vi "Noise-Create.vi"(4 "Rep Num":i32, 6 "Name":string, 8 "error in (no error)":errorcluster, 9 "Npts":i32, 10 "Sampling Rate (Hz)":dbl, 11 "Noise Params":T1) -> (0 "error out":errorcluster, 2 "Waveform":dbl[](array[numeric]), 3 "Noise Params (out)":T1)   [LabVIEW 2020]
uses:
  Noise Params.ctl
  Noise-Globals.vi
  <vilib>/Analysis/NI_AALBase.lvlib
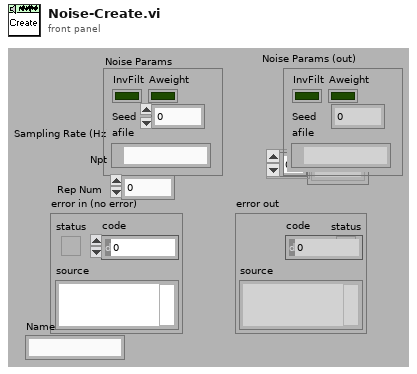
[diagram p1: front panel]
types:
  T1 = typedef "Noise Params.ctl" = cluster{"InvFilt":bool, "Noise":dbl[], "CurPt":i32, "Aweight":bool, "Seed":i32, "afile":path}
  T2 = enum16{"Clear", "Set data", "Reset index", "Get data"}
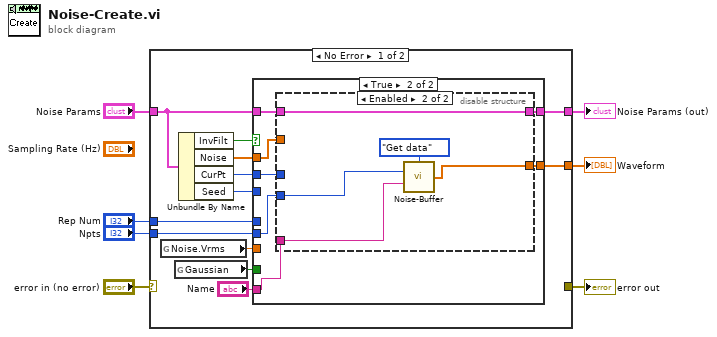
[diagram p0: block diagram]
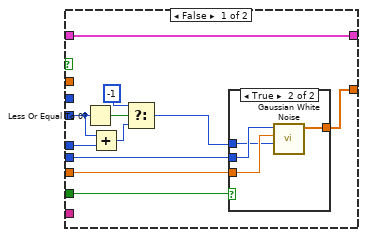
[diagram p2: hidden frame]
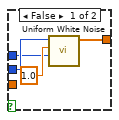
[diagram p3: hidden frame]
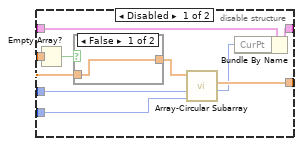
[diagram p4: hidden frame]
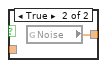
[diagram p5: hidden frame]
diagram:
  n1 = case shown="No Error" "error in (no error)" {
    selector: "error in (no error)" -> [_ w63]
    tunnel: "Npts" -> [w19 _]
    tunnel: [w18 _] -> w6
    tunnel: [_ w63] -> w4
    tunnel: [w15 w62] -> w2
    tunnel: "Noise Params" -> [w16 w62]
    tunnel: "Rep Num" -> [w9 _]
    frame No Error {
      n2 = global read "Noise-Globals.vi" "Noise.Vrms"() -> (w13:dbl)
      n3 = global read "Noise-Globals.vi" "Gaussian"() -> (w14:bool)
      n4 = Unbundle By Name(w16) -> ("InvFilt"=w8:bool, "Noise"=w12:dbl[], "CurPt"=w17:i32, "Seed"=w10:i32)
      n5 = case shown="True" w8 {
        tunnel: w19 -> [w22 w44]
        tunnel: [w30 w45] -> w18
        tunnel: w17 -> [_ w43]
        tunnel: w16 -> [w29 w42]
        tunnel: [w29 w41] -> w15
        tunnel: w14 -> [w28 _]
        tunnel: w13 -> [w27 _]
        tunnel: w12 -> [_ w40]
        tunnel: "Name" -> [_ w39]
        tunnel: w10 -> [w20 _]
        tunnel: w9 -> [w23 _]
        frame False {
          n6 = Less Or Equal To 0?(x=w20) -> (x <= 0?=w26:bool)
          n7 = Add(x=w20, y=w23) -> (x+y=w21:i32)
          n8 = Select(t=-1, s=w26, f=w21) -> (s? t:f=w24:i32)
          n9 = case shown="True" w28 {
            tunnel: w22 -> [w34 w37]
            tunnel: [w33 w38] -> w30
            tunnel: w27 -> [_ w36]
            tunnel: w24 -> [w31 w35]
            frame False {
              n10 = call <vilib>:"Uniform White Noise.vi"("seed"=w31, "amplitude"=1.0, "samples"=w34) -> ("uniform white noise"=w33:dbl[])  [unwired: 7 in, 1 out]
            }
            frame True {
              n11 = call <vilib>:"Gaussian White Noise.vi"("seed"=w35, "standard deviation"=w36, "samples"=w37) -> ("Gaussian noise pattern"=w38:dbl[])  [unwired: 7 in, 1 out]
            }
          }
        }
        frame True {
          n12 = disable-structure shown="Enabled" {
            disable-tunnel: [w54 w59] -> w45
            disable-tunnel: w44 -> [w53 w60]
            disable-tunnel: w43 -> [w52 _]
            disable-tunnel: w42 -> [w51 w57]
            disable-tunnel: [w50 w57] -> w41
            disable-tunnel: w40 -> [w46 _]
            disable-tunnel: w39 -> [_ w61]
            frame Disabled {
              n13 = Empty Array?(array=w46) -> (empty?=w48:bool)
              n14 = case shown="False" w48 {
                tunnel: [w55 w56] -> w47
                tunnel: w46 -> [w55 _]
                frame False {
                }
                frame True {
                  n15 = global read "Noise-Globals.vi" "Noise"() -> (w56:dbl[])
                }
              }
              n16 = call "Array-Circular Subarray.vi"("Npts"=w53, "Offset (in)"=w52, "Array"=w47) -> ("Offset (out)"=w49:i32, "Subarray"=w54:dbl[])  [unwired: 7 in]
              n17 = Bundle By Name(cluster=w51, "CurPt"=w49) -> (w50:T1)
            }
            frame Enabled {
              n18 = call "Noise-Buffer.vi"("Action"=T2."Get data", "Npts"=w60, "Name"=w61) -> ("Data Out"=w59:dbl[])  [unwired: 11 in, 1 out]
            }
          }
        }
      }
    }
    frame Error {
    }
  }
  "error out" <- w4
  "Waveform" <- w6
  "Noise Params (out)" <- w2
